vi "DrawEllipseEquispacedPoints.vi"(8 "Phase":dbl, 9 "Eccentricity":dbl, 10 "Radius":dbl, 11 "Points":i32) -> (3 "Array":dbl[](array[numeric]))   [LabVIEW 2017]
uses:
  AODControl/AODControl.lvlib
panel:
  out "Array 6":dbl[](array[numeric])
  out "Array 5":dbl[](array[numeric])
  out "Array 4":dbl[](array[numeric])
  out "Array 3":dbl[](array[numeric])
  out "Distance":dbl
  out "Array 2":dbl[](array[numeric])
  out "Ds 2":dbl
  out "(Ds)' 2":dbl
  out "Dt":dbl
  out "(Ds)'":dbl
  out "Ds":dbl
  out "a":dbl
  out "b":dbl
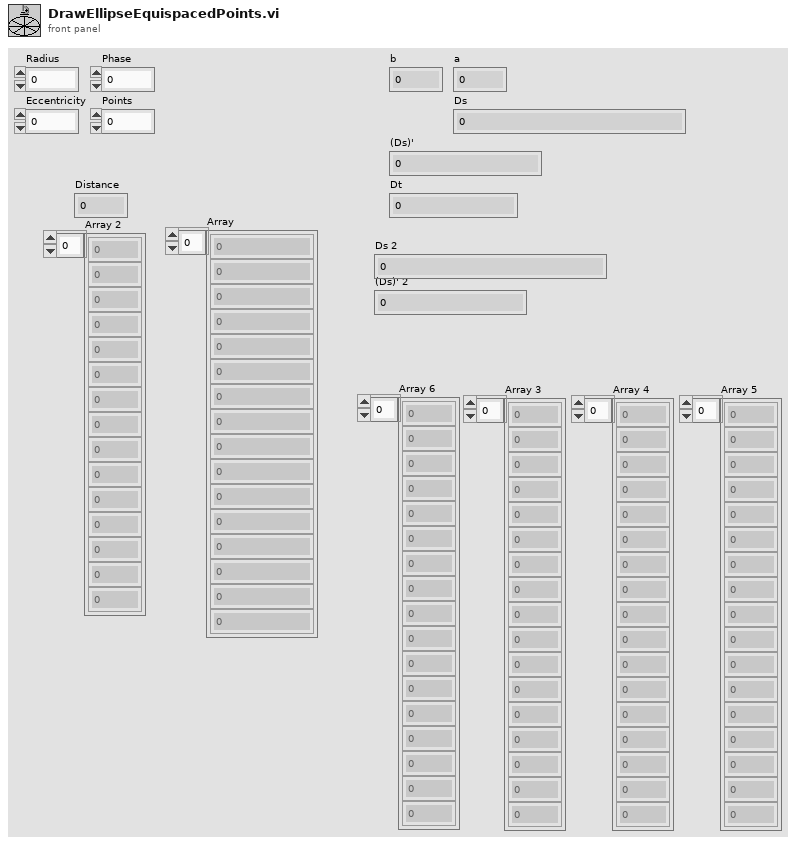
[diagram p1: front panel]
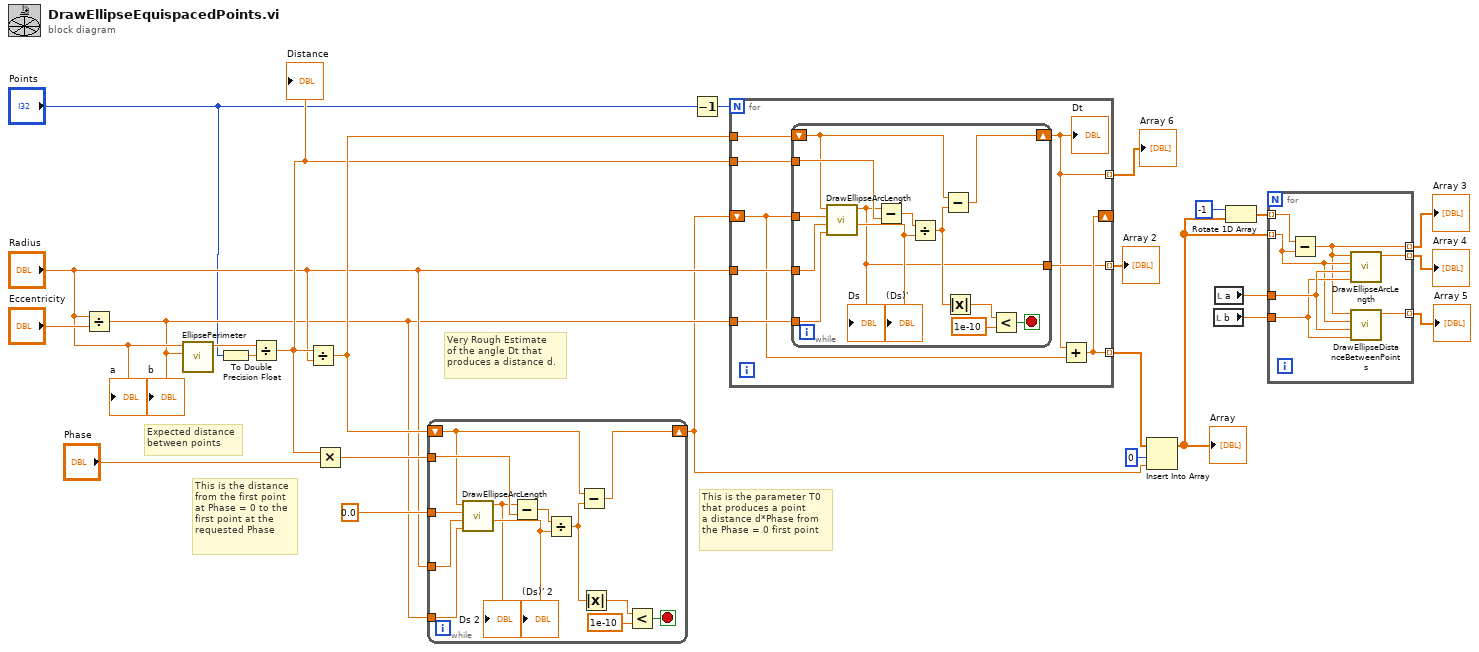
[diagram p0: block diagram]
diagram:
  # "This is the parameter T0 \nthat produces a point \na distance d*Phase from\nthe Phase = 0 first point"
  # "This is the distance\nfrom the first point\nat Phase = 0 to the \nfirst point at the \nrequested Phase"
  # "Very Rough Estimate\nof the angle Dt that \nproduces a distance d."
  # "Expected distance\nbetween points"
  n1 = Divide ("b")(x="Radius", y="Eccentricity") -> (x/y=w16:dbl)
  "b" <- w16
  n2 = call "EllipsePerimeter.vi"("a"=w16, "b"="Radius") -> ("Numeric"=w24:dbl)  [unwired: 9 in]
  n3 = To Double Precision Float(number="Points") -> (double precision float=w23:dbl)
  n4 = Divide(x=w24, y=w23) -> (x/y=w21:dbl)
  "Distance" <- w21
  n5 = Divide ("Dt Estimate")(x=w21, y="Radius") -> (x/y=w22:dbl)
  n6 = Multiply(x=w21, y="Phase") -> (x*y=w19:dbl)
  n7 = while {
    tunnel: 0.0 ("T0") -> [w32]
    tunnel: w16 -> [w30]
    tunnel: "Radius" -> [w31]
    shift-right: [w38] -> w11
    shift-left: w22 -> [w27]
    tunnel: w19 -> [w37]
    stop <- w33 stop-if-true
    n8 = call "DrawEllipseArcLength.vi"("b"=w30, "a"=w31, "t"=w32, "Dt"=w27) -> ("Ds'"=w28:dbl, "Ds"=w26:dbl)  [unwired: 6 in]
    "Ds 2" <- w26
    "(Ds)' 2" <- w28
    n9 = Subtract(x=w26, y=w37) -> (x-y=w29:dbl)
    n10 = Divide(x=w29, y=w28) -> (x/y=w36:dbl)
    n11 = Subtract(x=w27, y=w36) -> (x-y=w38:dbl)
    n12 = Absolute Value(x=w36) -> (abs(x)=w35:dbl)
    n13 = Less?(x=w35, y=1e-10) -> (x < y?=w33:bool)
  }
  n14 = Decrement(x="Points") -> (x-1=w14:i32)
  n15 = for {
    N: w14 -> [_]
    tunnel: w16 -> [w46]
    tunnel: "Radius" -> [w45]
    tunnel: w22 -> [w44]
    tunnel: w21 -> [w43]
    tunnel: [w42] -> w12 mode=indexing
    shift-right: [w42] -> _
    shift-left: w11 -> [w41]
    tunnel: [w40] -> w15 mode=indexing
    tunnel: [w39] -> w4 mode=indexing
    n16 = while {
      tunnel: w41 -> [w53]
      tunnel: w46 -> [w51]
      tunnel: w45 -> [w52]
      shift-right: [w59] -> w39
      shift-left: w44 -> [w48]
      tunnel: w43 -> [w58]
      tunnel: [w47] -> w40
      stop <- w54 stop-if-true
      n17 = call "DrawEllipseArcLength.vi"("b"=w51, "a"=w52, "t"=w53, "Dt"=w48) -> ("Ds'"=w49:dbl, "Ds"=w47:dbl)  [unwired: 6 in]
      "Ds" <- w47
      "(Ds)'" <- w49
      n18 = Subtract(x=w47, y=w58) -> (x-y=w50:dbl)
      n19 = Divide(x=w50, y=w49) -> (x/y=w57:dbl)
      n20 = Subtract(x=w48, y=w57) -> (x-y=w59:dbl)
      n21 = Absolute Value(x=w57) -> (abs(x)=w56:dbl)
      n22 = Less?(x=w56, y=1e-10) -> (x < y?=w54:bool)
    }
    "Dt" <- w39
    n23 = Add(x=w39, y=w41) -> (x+y=w42:dbl)
  }
  "Array 2" <- w15
  "Array 6" <- w4
  n24 = Insert Into Array(array=w12, index=0, new element=w11) -> (w2:dbl[])
  "Array" <- w2
  n25 = local read "b"() -> (w7:dbl)
  n26 = local read "a"() -> (w8:dbl)
  n27 = Rotate 1D Array(1:w2, 2:-1 ("n")) -> (0:w3:dbl[])
  n28 = for {
    tunnel: w3 -> [w61] mode=indexing
    tunnel: w2 -> [w62] mode=indexing
    tunnel: [w60] -> w9 mode=indexing
    tunnel: w8 -> [w66]
    tunnel: w7 -> [w65]
    tunnel: [w64] -> w5 mode=indexing
    tunnel: [w63] -> w6 mode=indexing
    n29 = Subtract(x=w61, y=w62) -> (x-y=w60:dbl)
    n30 = call "DrawEllipseArcLength.vi"("b"=w65, "a"=w66, "t"=w62, "Dt"=w60) -> ("Ds"=w63:dbl)  [unwired: 6 in, 1 out]
    n31 = call "DrawEllipseDistanceBetweenPoints.vi"("b"=w65, "a"=w66, "t"=w62, "Dt"=w60) -> ("Ds"=w64:dbl)  [unwired: 6 in, 1 out]
  }
  "Array 3" <- w9
  "Array 4" <- w6
  "Array 5" <- w5
  "a" <- "Radius"
